vi "BoP.vi"() -> ()   [LabVIEW 2017]
panel:
  in  "error in (no error)":errorcluster
  out "Time":sgl
  in  "LPT PR":sgl=0.2 min=0.1 max=0.9 step=0.001 format="%.3f"
  in  "HPT PR":sgl=0.278 min=0.1 max=0.9 step=0.001 format="%.3f"
  in  "NG Press":sgl=45.0 min=1 max=50 step=0.1 format="%.1f"
  in  "NG Temp":sgl=75.0 min=0 max=80 step=0.1 format="%.1f"
  in  "Air Flow Rate":sgl=418.0 min=1 max=500 step=0.1
  out "h7":sgl format="%.1f"
  out "h6":sgl format="%.1f"
  out "h5":sgl format="%.1f"
  out "h4":sgl format="%.1f"
  out "h3":sgl format="%.1f"
  out "h2":sgl format="%.1f"
  out "h1":sgl format="%.1f"
  out "mdot1":sgl format="%.1f"
  out "P1":sgl format="%.1f"
  out "T1":sgl format="%.1f"
  out "mdot7":sgl format="%.1f"
  out "mdot6":sgl format="%.1f"
  out "mdot5":sgl format="%.1f"
  out "mdot4":sgl format="%.1f"
  out "mdot3":sgl format="%.1f"
  out "mdot2":sgl format="%.1f"
  out "P5":sgl format="%.1f"
  out "T5":sgl format="%.1f"
  in  "Stop":bool
  in  "NG Flow Rate":sgl min=0 max=10 step=0.01 format="%.2f"
  out "LP CTAH Heat In":sgl=418.0 format="%_3f"
  out "HP CTAH Heat In":sgl=418.0 format="%_3f"
  out "Compressor Work":sgl=1000000.0 format="%_3f"
  in  "Shaft RPM":sgl=3600.0 min=0 max=3600 step=1
  out "Mass Flow":cluster{"Single":sgl, "Single":sgl}(graph)
  out "Turbine Work Output":cluster{"Single":sgl, "Single":sgl}(graph)
  out "P2":sgl format="%.1f"
  out "T2":sgl format="%.1f"
  out "P3":sgl format="%.1f"
  out "T3":sgl format="%.1f"
  out "P4":sgl format="%.1f"
  out "T4":sgl format="%.1f"
  out "P6":sgl format="%.1f"
  out "T6":sgl format="%.1f"
  out "P7":sgl format="%.1f"
  out "T7":sgl format="%.1f"
  out "HPT Work Out":sgl=1000000.0 format="%_3f"
  out "LPT Work Out":sgl=137940000.0 format="%_3f"
  out "Pressure Drop 1st Pass":sgl
  out "Pressure Drop 2nd pass":sgl
  # "Balance of Plant"
  # "Trends and Analytics"
  # "LPT Out"
  # "Compressor In"
  # "C"
  # "bar"
  # "C"
  # "bar"
  # "kg/s"
  # "MW"
  # "kg/s"
  # "MW"
  # "HIGH PRESSURE\nTURBINE"
  # "LOW PRESSURE\nTURBINE"
  # "COMPRESSOR"
  # "Compressor Out"
  # "C"
  # "bar"
  # "kg/s"
  # "MW"
  # "CTAH"
  # "HP CTAH Out"
  # "C"
  # "bar"
  # "HPT Out"
  # "kg/s"
  # "MW"
  # "C"
  # "bar"
  # "kg/s"
  # "MW"
  # "Combustor Out"
  # "C"
  # "bar"
  # "kg/s"
  # "MW"
  # "COMBUSTOR"
  # "LP CTAH Out"
  # "C"
  # "bar"
  # "kg/s"
  # "MW"
  # "Load and Demand"
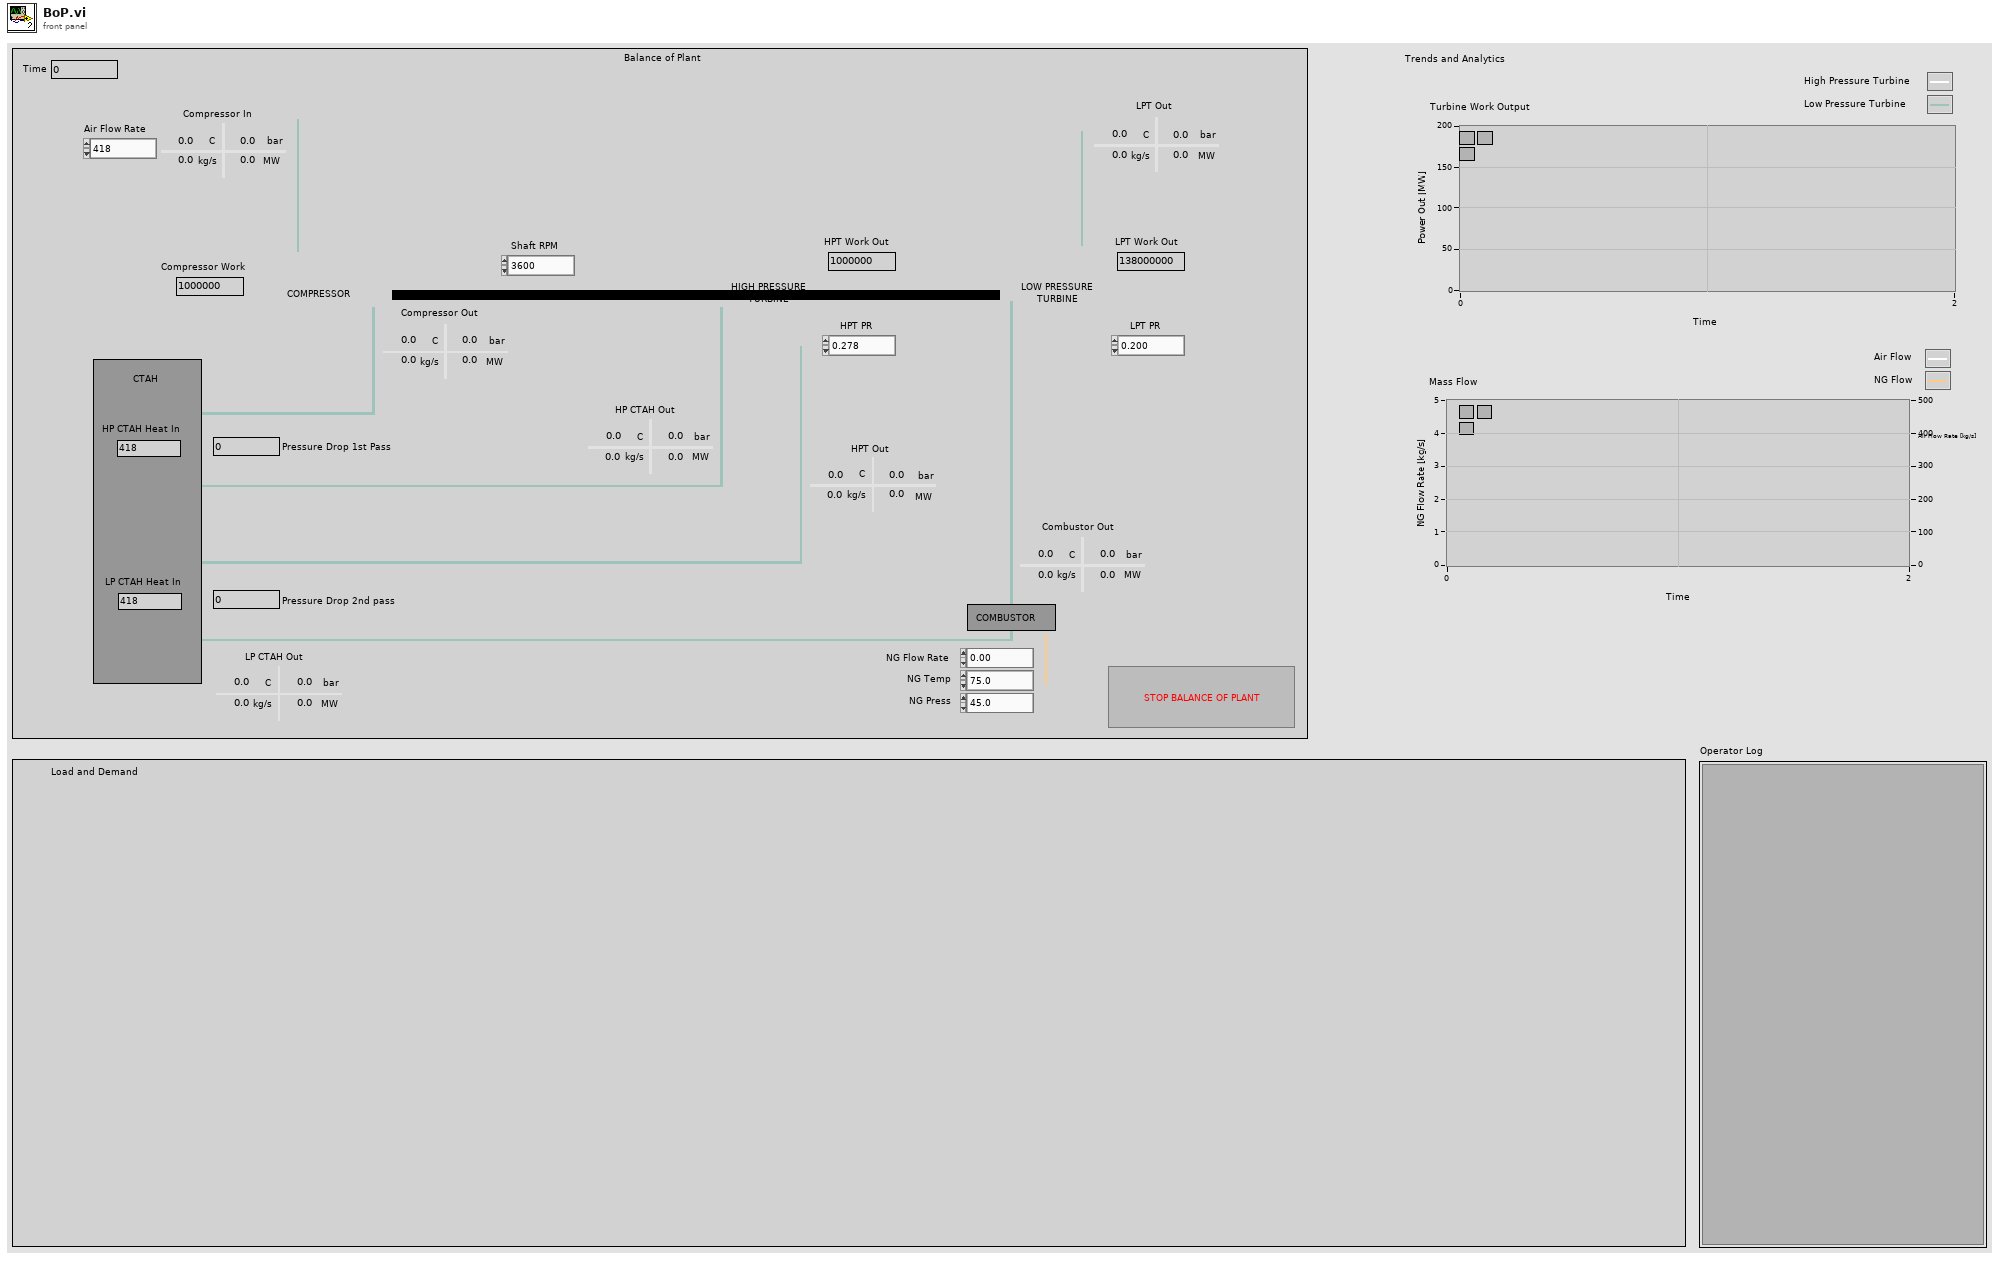
[diagram p1: front panel]
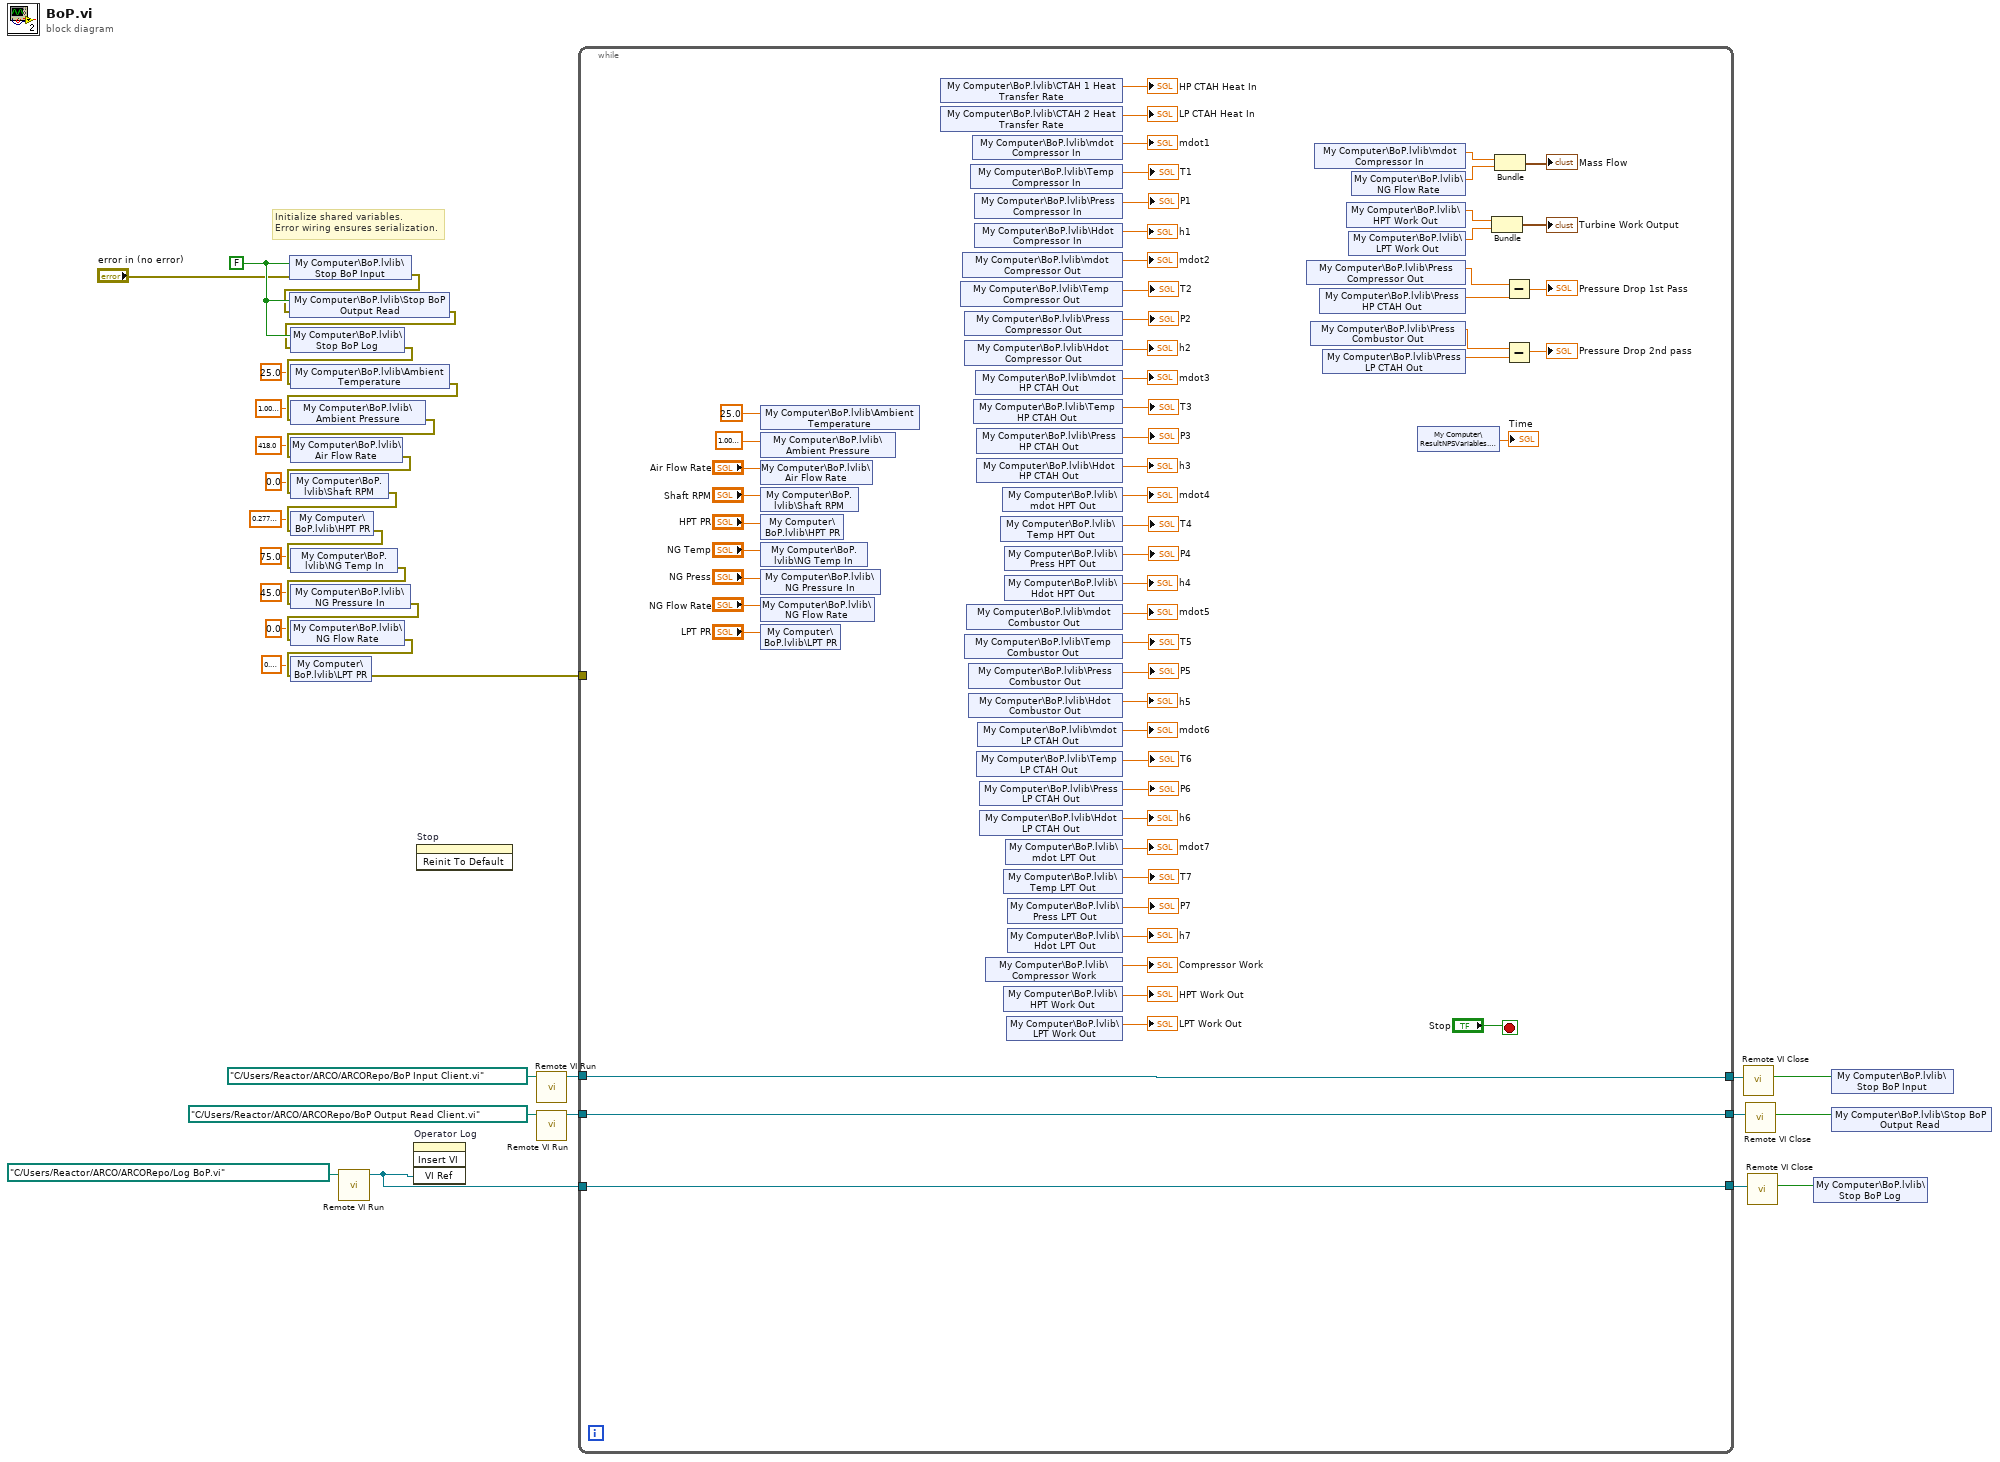
[diagram p0: block diagram]
diagram:
  w23 = FALSE
  # "Initialize shared variables.\nError wiring ensures serialization."
  n1 = shared-variable "My Computer\\BoP.lvlib\\Stop BoP Input"(w23, error in="error in (no error)") -> (error out=w22:errorcluster)
  n2 = shared-variable "My Computer\\BoP.lvlib\\Stop BoP Output Read"(w23, error in=w22) -> (error out=w20:errorcluster)
  n3 = shared-variable "My Computer\\BoP.lvlib\\Stop BoP Log"(w23, error in=w20) -> (error out=w21:errorcluster)
  n4 = shared-variable "My Computer\\BoP.lvlib\\Ambient Temperature"(sgl 25.0 ("Ambient Temperature"), error in=w21) -> (error out=w19:errorcluster)
  n5 = shared-variable "My Computer\\BoP.lvlib\\Ambient Pressure"(sgl 1.01 ("Ambient Pressure"), error in=w19) -> (error out=w18:errorcluster)
  n6 = shared-variable "My Computer\\BoP.lvlib\\Air Flow Rate"(sgl 418.0 ("Air Flow Rate"), error in=w18) -> (error out=w17:errorcluster)
  n7 = shared-variable "My Computer\\BoP.lvlib\\Shaft RPM"(sgl 0.0 ("Shaft RPM"), error in=w17) -> (error out=w16:errorcluster)
  n8 = shared-variable "My Computer\\BoP.lvlib\\HPT PR"(sgl 0.278 ("HPT PR"), error in=w16) -> (error out=w15:errorcluster)
  n9 = shared-variable "My Computer\\BoP.lvlib\\NG Temp In"(sgl 75.0 ("NG Temp In"), error in=w15) -> (error out=w14:errorcluster)
  n10 = shared-variable "My Computer\\BoP.lvlib\\NG Pressure In"(sgl 45.0 ("NG Pressure In"), error in=w14) -> (error out=w13:errorcluster)
  n11 = shared-variable "My Computer\\BoP.lvlib\\NG Flow Rate"(sgl 0.0 ("NG Flow Rate"), error in=w13) -> (error out=w12:errorcluster)
  n12 = shared-variable "My Computer\\BoP.lvlib\\LPT PR"(sgl 0.2 ("LPT PR"), error in=w12) -> (error out=w2:errorcluster)
  n13 = call "Remote VI Run.vi"("VI Path"=path "C:/Users/Reactor/ARCO/ARCORepo/Log BoP.vi" ("vi path")) -> ("VI Reference"=w27:refnum<vi>)  [unwired: 10 in]
  n14 = invoke on="Operator Log" class="SubPnl" method="Insert VI"("VI Ref"=w27) -> ()  [unwired: 3 in, 4 out]
  n15 = invoke on="Stop" class="Bool" method="Reinit To Default"() -> ()  [unwired: 3 in, 3 out]
  n16 = call "Remote VI Run.vi"("VI Path"=path "C:/Users/Reactor/ARCO/ARCORepo/BoP Input Client.vi") -> ("VI Reference"=w35:refnum<vi>)  [unwired: 10 in]
  n17 = call "Remote VI Run.vi"("VI Path"=path "C:/Users/Reactor/ARCO/ARCORepo/BoP Output Read Client.vi") -> ("VI Reference"=w33:refnum<vi>)  [unwired: 10 in]
  n18 = while {
    tunnel: w35 -> [w49]
    tunnel: [w49] -> w34
    tunnel: w33 -> [w48]
    tunnel: [w48] -> w32
    tunnel: [w47] -> w28
    tunnel: w27 -> [w47]
    tunnel: w2 -> [_]
    stop <- "Stop" stop-if-true
    n19 = shared-variable "My Computer\\BoP.lvlib\\Ambient Temperature"(sgl 25.0 ("Incoming Air Temp")) -> ()  [unwired: 1 in, 1 out]
    n20 = shared-variable "My Computer\\BoP.lvlib\\Ambient Pressure"(sgl 1.01 ("Incoming Air Pressure")) -> ()  [unwired: 1 in, 1 out]
    n21 = shared-variable "My Computer\\BoP.lvlib\\Air Flow Rate"("Air Flow Rate") -> ()  [unwired: 1 in, 1 out]
    n22 = shared-variable "My Computer\\BoP.lvlib\\Shaft RPM"("Shaft RPM") -> ()  [unwired: 1 in, 1 out]
    n23 = shared-variable "My Computer\\BoP.lvlib\\HPT PR"("HPT PR") -> ()  [unwired: 1 in, 1 out]
    n24 = shared-variable "My Computer\\BoP.lvlib\\NG Temp In"("NG Temp") -> ()  [unwired: 1 in, 1 out]
    n25 = shared-variable "My Computer\\BoP.lvlib\\NG Pressure In"("NG Press") -> ()  [unwired: 1 in, 1 out]
    n26 = shared-variable "My Computer\\BoP.lvlib\\NG Flow Rate"("NG Flow Rate") -> ()  [unwired: 1 in, 1 out]
    n27 = shared-variable "My Computer\\BoP.lvlib\\LPT PR"("LPT PR") -> ()  [unwired: 1 in, 1 out]
    n28 = shared-variable "My Computer\\BoP.lvlib\\CTAH 1 Heat Transfer Rate"() -> (→"HP CTAH Heat In":sgl)  [unwired: 1 in, 1 out]
    n29 = shared-variable "My Computer\\BoP.lvlib\\CTAH 2 Heat Transfer Rate"() -> (→"LP CTAH Heat In":sgl)  [unwired: 1 in, 1 out]
    n30 = shared-variable "My Computer\\BoP.lvlib\\Temp Compressor Out"() -> (→"T2":sgl)  [unwired: 1 in, 1 out]
    n31 = shared-variable "My Computer\\BoP.lvlib\\mdot Compressor Out"() -> (→"mdot2":sgl)  [unwired: 1 in, 1 out]
    n32 = shared-variable "My Computer\\BoP.lvlib\\Press Compressor Out"() -> (→"P2":sgl)  [unwired: 1 in, 1 out]
    n33 = shared-variable "My Computer\\BoP.lvlib\\Hdot Compressor Out"() -> (→"h2":sgl)  [unwired: 1 in, 1 out]
    n34 = shared-variable "My Computer\\BoP.lvlib\\Temp Combustor Out"() -> (→"T5":sgl)  [unwired: 1 in, 1 out]
    n35 = shared-variable "My Computer\\BoP.lvlib\\mdot Combustor Out"() -> (→"mdot5":sgl)  [unwired: 1 in, 1 out]
    n36 = shared-variable "My Computer\\BoP.lvlib\\Press Combustor Out"() -> (→"P5":sgl)  [unwired: 1 in, 1 out]
    n37 = shared-variable "My Computer\\BoP.lvlib\\Hdot Combustor Out"() -> (→"h5":sgl)  [unwired: 1 in, 1 out]
    n38 = shared-variable "My Computer\\BoP.lvlib\\Temp Compressor In"() -> (→"T1":sgl)  [unwired: 1 in, 1 out]
    n39 = shared-variable "My Computer\\BoP.lvlib\\mdot Compressor In"() -> (→"mdot1":sgl)  [unwired: 1 in, 1 out]
    n40 = shared-variable "My Computer\\BoP.lvlib\\Temp HP CTAH Out"() -> (→"T3":sgl)  [unwired: 1 in, 1 out]
    n41 = shared-variable "My Computer\\BoP.lvlib\\Press Compressor In"() -> (→"P1":sgl)  [unwired: 1 in, 1 out]
    n42 = shared-variable "My Computer\\BoP.lvlib\\Hdot Compressor In"() -> (→"h1":sgl)  [unwired: 1 in, 1 out]
    n43 = shared-variable "My Computer\\BoP.lvlib\\mdot HP CTAH Out"() -> (→"mdot3":sgl)  [unwired: 1 in, 1 out]
    n44 = shared-variable "My Computer\\BoP.lvlib\\Temp LP CTAH Out"() -> (→"T6":sgl)  [unwired: 1 in, 1 out]
    n45 = shared-variable "My Computer\\BoP.lvlib\\Press HP CTAH Out"() -> (→"P3":sgl)  [unwired: 1 in, 1 out]
    n46 = shared-variable "My Computer\\BoP.lvlib\\Hdot HP CTAH Out"() -> (→"h3":sgl)  [unwired: 1 in, 1 out]
    n47 = shared-variable "My Computer\\BoP.lvlib\\mdot LP CTAH Out"() -> (→"mdot6":sgl)  [unwired: 1 in, 1 out]
    n48 = shared-variable "My Computer\\BoP.lvlib\\Press LP CTAH Out"() -> (→"P6":sgl)  [unwired: 1 in, 1 out]
    n49 = shared-variable "My Computer\\BoP.lvlib\\Hdot LP CTAH Out"() -> (→"h6":sgl)  [unwired: 1 in, 1 out]
    n50 = shared-variable "My Computer\\BoP.lvlib\\Compressor Work"() -> (→"Compressor Work":sgl)  [unwired: 1 in, 1 out]
    n51 = shared-variable "My Computer\\BoP.lvlib\\Temp HPT Out"() -> (→"T4":sgl)  [unwired: 1 in, 1 out]
    n52 = shared-variable "My Computer\\BoP.lvlib\\mdot HPT Out"() -> (→"mdot4":sgl)  [unwired: 1 in, 1 out]
    n53 = shared-variable "My Computer\\BoP.lvlib\\Temp LPT Out"() -> (→"T7":sgl)  [unwired: 1 in, 1 out]
    n54 = shared-variable "My Computer\\BoP.lvlib\\HPT Work Out"() -> (→"HPT Work Out":sgl)  [unwired: 1 in, 1 out]
    n55 = shared-variable "My Computer\\BoP.lvlib\\Press HPT Out"() -> (→"P4":sgl)  [unwired: 1 in, 1 out]
    n56 = shared-variable "My Computer\\BoP.lvlib\\Hdot HPT Out"() -> (→"h4":sgl)  [unwired: 1 in, 1 out]
    n57 = shared-variable "My Computer\\BoP.lvlib\\mdot LPT Out"() -> (→"mdot7":sgl)  [unwired: 1 in, 1 out]
    n58 = shared-variable "My Computer\\BoP.lvlib\\LPT Work Out"() -> (→"LPT Work Out":sgl)  [unwired: 1 in, 1 out]
    n59 = shared-variable "My Computer\\BoP.lvlib\\Press LPT Out"() -> (→"P7":sgl)  [unwired: 1 in, 1 out]
    n60 = shared-variable "My Computer\\BoP.lvlib\\Hdot LPT Out"() -> (→"h7":sgl)  [unwired: 1 in, 1 out]
    n61 = shared-variable "My Computer\\BoP.lvlib\\Press Compressor Out"() -> (w57:sgl)  [unwired: 1 in, 1 out]
    n62 = shared-variable "My Computer\\BoP.lvlib\\Press Combustor Out"() -> (w55:sgl)  [unwired: 1 in, 1 out]
    n63 = shared-variable "My Computer\\BoP.lvlib\\mdot Compressor In"() -> (w42:sgl)  [unwired: 1 in, 1 out]
    n64 = shared-variable "My Computer\\BoP.lvlib\\Press HP CTAH Out"() -> (w56:sgl)  [unwired: 1 in, 1 out]
    n65 = shared-variable "My Computer\\BoP.lvlib\\Press LP CTAH Out"() -> (w54:sgl)  [unwired: 1 in, 1 out]
    n66 = shared-variable "My Computer\\BoP.lvlib\\HPT Work Out"() -> (w38:sgl)  [unwired: 1 in, 1 out]
    n67 = shared-variable "My Computer\\BoP.lvlib\\LPT Work Out"() -> (w37:sgl)  [unwired: 1 in, 1 out]
    n68 = shared-variable "My Computer\\BoP.lvlib\\NG Flow Rate"() -> (w41:sgl)  [unwired: 1 in, 1 out]
    n69 = shared-variable "My Computer\\ResultNPSVariables.lvlib\\Time_R"() -> (→"Time":sgl)  [unwired: 1 in, 1 out]
    n70 = Bundle("Single"=w38, "Single"=w37) -> (→"Turbine Work Output":cluster{"Single":sgl, "Single":sgl})  [unwired: 1 in]
    n71 = Bundle("Single"=w42, "Single"=w41) -> (→"Mass Flow":cluster{"Single":sgl, "Single":sgl})  [unwired: 1 in]
    n72 = Subtract(x=w57, y=w56) -> (x-y=→"Pressure Drop 1st Pass":sgl)
    n73 = Subtract(x=w55, y=w54) -> (x-y=→"Pressure Drop 2nd pass":sgl)
  }
  n74 = call "Remote VI Close.vi"("reference"=w34) -> ("SubVI Stop"=w26:bool)  [unwired: 10 in]
  n75 = call "Remote VI Close.vi"("reference"=w32) -> ("SubVI Stop"=w25:bool)  [unwired: 10 in]
  n76 = call "Remote VI Close.vi"("reference"=w28) -> ("SubVI Stop"=w24:bool)  [unwired: 10 in]
  n77 = shared-variable "My Computer\\BoP.lvlib\\Stop BoP Log"(w24) -> ()  [unwired: 1 in, 1 out]
  n78 = shared-variable "My Computer\\BoP.lvlib\\Stop BoP Input"(w26) -> ()  [unwired: 1 in, 1 out]
  n79 = shared-variable "My Computer\\BoP.lvlib\\Stop BoP Output Read"(w25) -> ()  [unwired: 1 in, 1 out]
